vi "output.vi"(8 "error in":errorcluster, 10 "data table in":T1, 11 "CVT runtime in":refnum<class "CVT runtime.lvclass">) -> (0 "error out":errorcluster, 2 "data table out":T1, 3 "CVT runtime out":refnum<class "CVT runtime.lvclass">)   [LabVIEW 2013, in "CVT runtime.lvclass"]
doc: "Provides an interface for writing data to a module at runtime. While this interface performs no operations, a child should provide an override which may write to any open sessions, references, or interfaces."
uses:
  CVT runtime.lvclass
  <vilib>/NI/Tag Bus/table/data table.ctl
  CVT runtime.lvclass/CVT runtime.ctl
  <vilib>/NI/Current Value Table/Write Index Set.vi
  <vilib>/NI/Current Value Table/DataTypes/Double_Write Index Set.vi
  <vilib>/NI/Current Value Table/DataTypes/Array of String_Write Index Set.vi
  <vilib>/NI/Current Value Table/DataTypes/Array of Boolean_Write Index Set.vi
  <vilib>/NI/Current Value Table/DataTypes/Array of Single_Write Index Set.vi
  <vilib>/NI/Current Value Table/DataTypes/Array of Double_Write Index Set.vi
  <vilib>/NI/Current Value Table/DataTypes/Array of I8_Write Index Set.vi
  <vilib>/NI/Current Value Table/DataTypes/Array of I16_Write Index Set.vi
  <vilib>/NI/Current Value Table/DataTypes/Array of I32_Write Index Set.vi
  <vilib>/NI/Current Value Table/DataTypes/Array of I64_Write Index Set.vi
  <vilib>/NI/Current Value Table/DataTypes/Array of U64_Write Index Set.vi
  <vilib>/NI/Current Value Table/DataTypes/Array of U32_Write Index Set.vi
  <vilib>/NI/Current Value Table/DataTypes/Array of U16_Write Index Set.vi
  <vilib>/NI/Current Value Table/DataTypes/Array of U8_Write Index Set.vi
  <vilib>/NI/Current Value Table/DataTypes/Boolean_Write Index Set.vi
  <vilib>/NI/Current Value Table/DataTypes/String_Write Index Set.vi
  <vilib>/NI/Current Value Table/DataTypes/U8_Write Index Set.vi
  <vilib>/NI/Current Value Table/DataTypes/U16_Write Index Set.vi
  <vilib>/NI/Current Value Table/DataTypes/U32_Write Index Set.vi
  <vilib>/NI/Current Value Table/DataTypes/U64_Write Index Set.vi
  <vilib>/NI/Current Value Table/DataTypes/I8_Write Index Set.vi
  <vilib>/NI/Current Value Table/DataTypes/I16_Write Index Set.vi
  <vilib>/NI/Current Value Table/DataTypes/I32_Write Index Set.vi
  <vilib>/NI/Current Value Table/DataTypes/I64_Write Index Set.vi
  <vilib>/NI/Current Value Table/DataTypes/Single_Write Index Set.vi
  <vilib>/NI/Current Value Table/Memory Block.vi
  <vilib>/NI/Current Value Table/DataTypes/Double_Memory Block.vi
  <vilib>/NI/Current Value Table/DataTypes/Array of String_Memory Block.vi
  <vilib>/NI/Current Value Table/DataTypes/Array of Boolean_Memory Block.vi
  <vilib>/NI/Current Value Table/DataTypes/Array of Single_Memory Block.vi
  <vilib>/NI/Current Value Table/DataTypes/Array of Double_Memory Block.vi
  <vilib>/NI/Current Value Table/DataTypes/Array of I8_Memory Block.vi
  <vilib>/NI/Current Value Table/DataTypes/Array of I16_Memory Block.vi
  <vilib>/NI/Current Value Table/DataTypes/Array of I32_Memory Block.vi
  <vilib>/NI/Current Value Table/DataTypes/Array of I64_Memory Block.vi
  <vilib>/NI/Current Value Table/DataTypes/Array of U64_Memory Block.vi
  <vilib>/NI/Current Value Table/DataTypes/Array of U32_Memory Block.vi
  <vilib>/NI/Current Value Table/DataTypes/Array of U16_Memory Block.vi
  <vilib>/NI/Current Value Table/DataTypes/Array of U8_Memory Block.vi
  <vilib>/NI/Current Value Table/DataTypes/Boolean_Memory Block.vi
  <vilib>/NI/Current Value Table/DataTypes/String_Memory Block.vi
  <vilib>/NI/Current Value Table/DataTypes/U8_Memory Block.vi
  <vilib>/NI/Current Value Table/DataTypes/U16_Memory Block.vi
  <vilib>/NI/Current Value Table/DataTypes/U32_Memory Block.vi
  <vilib>/NI/Current Value Table/DataTypes/U64_Memory Block.vi
  <vilib>/NI/Current Value Table/DataTypes/I8_Memory Block.vi
  <vilib>/NI/Current Value Table/DataTypes/I16_Memory Block.vi
  <vilib>/NI/Current Value Table/DataTypes/I32_Memory Block.vi
  <vilib>/NI/Current Value Table/DataTypes/I64_Memory Block.vi
  <vilib>/NI/Current Value Table/DataTypes/Single_Memory Block.vi
  <vilib>/NI/Tag Bus/table/data table.lvlib
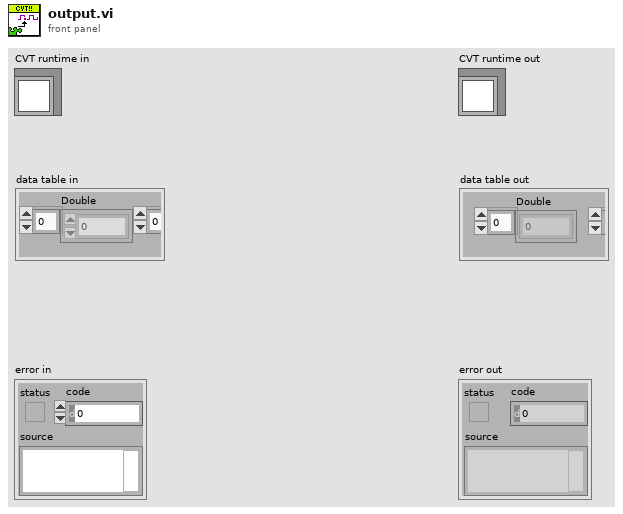
[diagram p1: front panel]
types:
  T1 = typedef "tag bus.lvlib/data table.lvlib/data table.ctl" = cluster{"Double":dbl[], "Single":sgl[], "I64":i64[], "I32":i32[], "I16":i16[], "I8":i8[], "U64":u64[], "U32":u32[], "U16":u16[], "U8":u8[], "Boolean":bool[], "String":string[], "Array of Double":cluster{"DBL Array":dbl[]}[], "Array of Single":cluster{"SGL Array":sgl[]}[], "Array of I64":cluster{"I64 Array":i64[]}[], "Array of I32":cluster{"I32 Array":i32[]}[], "Array of I16":cluster{"I16 Array":i16[]}[], "Array of I8":cluster{"I8 Array":i8[]}[], "Array of U64":cluster{"U64 Array":u64[]}[], "Array of U32":cluster{"U32 Array":u32[]}[], "Array of U16":cluster{"U16 Array":u16[]}[], "Array of U8":cluster{"U8 Array":u8[]}[], "Array of Boolean":cluster{"Boolean Array":bool[]}[], "Array of String":cluster{"String Array":string[]}[]}
  T2 = typedef "Current Value Table.lvlib/Typed Index Set.ctl" = cluster{"Data Type":T3, "Indices":i32[]}
  T3 = typedef "Current Value Table.lvlib/Data Types.ctl" = enum16{"Double", "Single", "I64", "I32", "I16", "I8", "U64", "U32", "U16", "U8", "String", "Boolean", "Array of U8", "Array of U16", "Array of U32", "Array of U64", "Array of I64", "Array of I32", "Array of I16", "Array of I8", "Array of Double", "Array of Single", "Array of Boolean", "Array of String"}
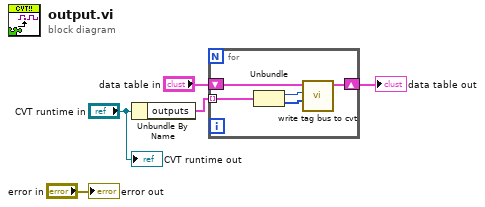
[diagram p0: block diagram]
diagram:
  n1 = Unbundle By Name("CVT runtime in") -> ("outputs"=w1:T2[])
  n2 = for {
    shift-right: [w10] -> w3
    shift-left: "data table in" -> [w9]
    tunnel: w1 -> [w8] mode=indexing
    n3 = Unbundle(w8) -> ("Data Type"=w7:T3, "Indices"=w6:i32[])
    n4 = call "write tag bus to cvt.vi"("Indices"=w6, "Data Type"=w7, "data table in"=w9) -> ("data table out"=w10:T1)  [unwired: 8 in]
  }
  "data table out" <- w3
  "error out" <- "error in"
  "CVT runtime out" <- "CVT runtime in"
